vi "BuildExperiment.vi"(0 "object in":refnum<class "Experiment.lvclass">, 1 "List of Frequencies":dbl[](array[numeric]) min=0.001, 2 "List of Amplitudes":dbl[](array[numeric]) min=0.001, 3 "Number of Images":i32, 4 "wait time(s)":dbl, 5 "error in (no error)":errorcluster, 7 "Flow":dbl[](array[numeric])) -> (14 "object out":refnum<class "Experiment.lvclass">, 17 "# elements in queue":i32, 19 "error out":errorcluster)   [LabVIEW 2023, in "Experiment.lvclass"]
uses:
  Experiment.lvclass
  Experiment.lvclass/Experiment.ctl
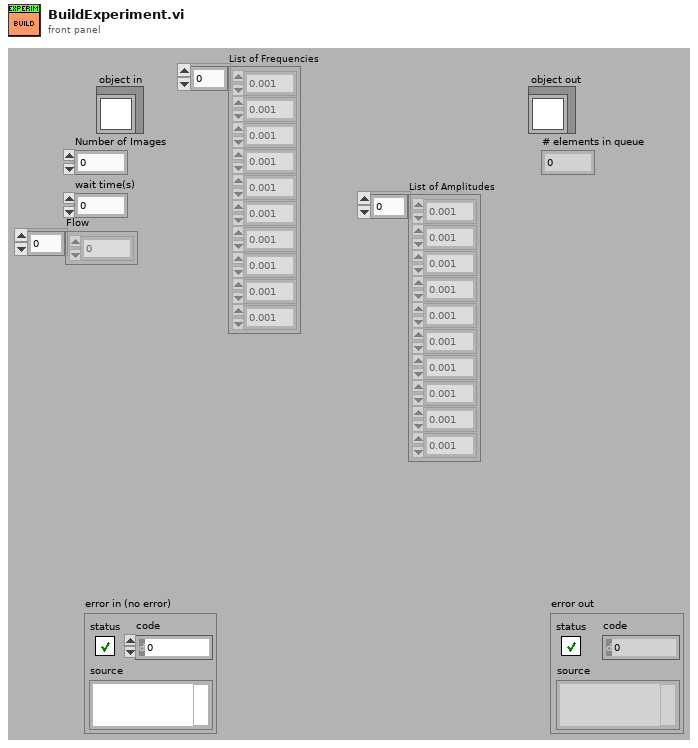
[diagram p1: front panel]
types:
  T1 = cluster{"index":i32, "Level(ml)":dbl, "Flow":dbl}
  T2 = cluster{"Enable Output WFG Ch1":bool, "Enable Output WFG Ch 2":bool}
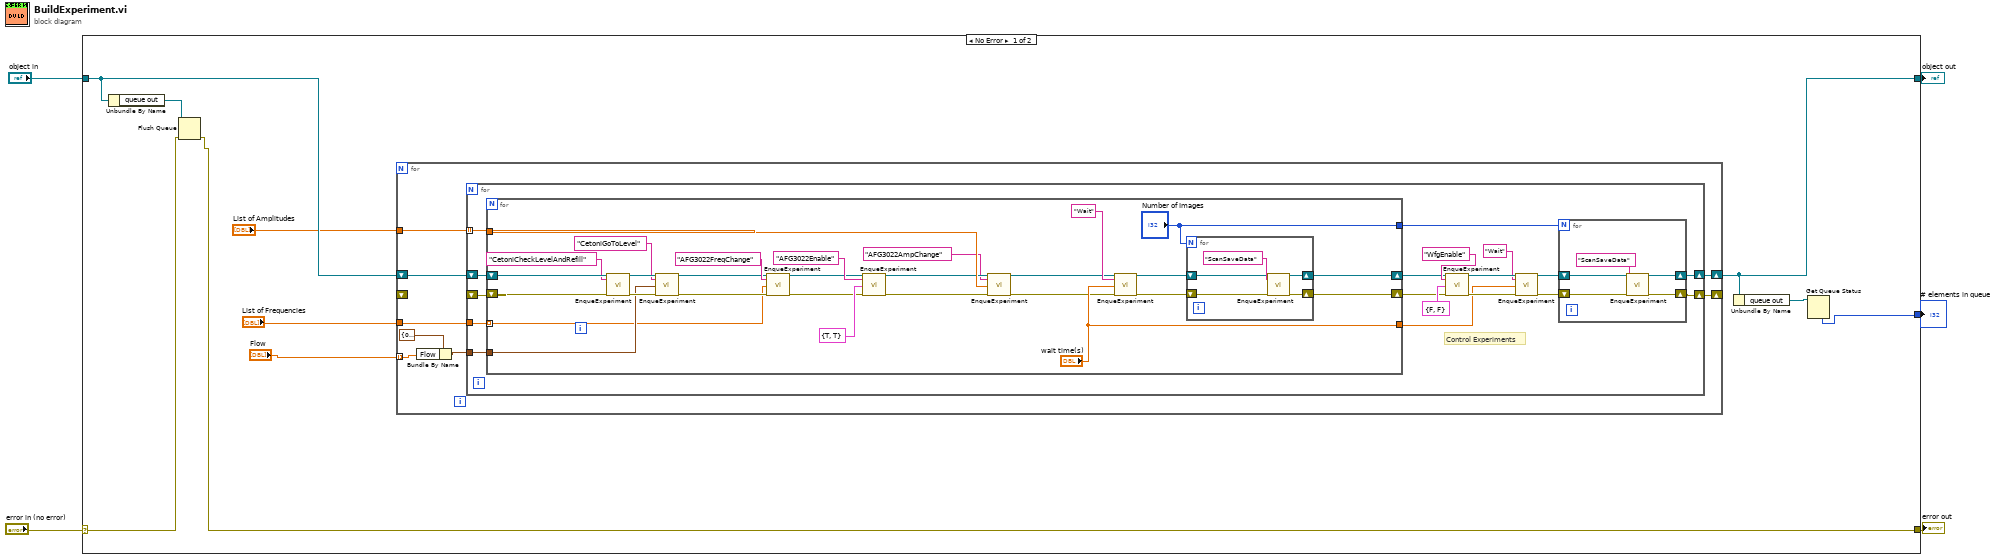
[diagram p0: block diagram]
diagram:
  n1 = case shown="No Error" "error in (no error)" {
    selector: "error in (no error)" -> [w12 w81]
    tunnel: [w11 w81] -> w4
    tunnel: [w10 w80] -> w2
    tunnel: "object in" -> [w14 w80]
    tunnel: [w8 _] -> w1
    frame No Error {
      n2 = Unbundle By Name(w14) -> ("queue out"=w13:refnum<queue>)
      n3 = Flush Queue(queue=w13, error in (no error)=w12) -> (error out=w11:errorcluster)  [unwired: 2 out]
      n4 = for {
        tunnel: "List of Frequencies" -> [w23]
        tunnel: "List of Amplitudes" -> [w20]
        shift-right: [w21] -> w10
        shift-left: w14 -> [w22]
        shift-right: [w19] -> _
        shift-left: _ -> [_]
        tunnel: "Flow" -> [w17] mode=indexing
        n5 = Bundle By Name(cluster=T1 {"index"=0, "Level(ml)"=0.0, "Flow"=0.0} ("GoToLevelSettings"), "Flow"=w17) -> (w16:T1)
        n6 = for {
          tunnel: w23 -> [w40]
          shift-right: [w31] -> w21
          shift-left: w22 -> [w39]
          tunnel: w20 -> [w41] mode=indexing
          tunnel: w16 -> [w25]
          shift-right: [w26] -> w19
          shift-left: _ -> [w24]
          # "Control Experiments"
          n7 = for {
            tunnel: w41 -> [w74]
            shift-right: [w65] -> w30
            shift-left: w39 -> [w63]
            tunnel: w40 -> [w50] mode=indexing
            tunnel: ["Number of Images"] -> w27
            shift-right: [w64] -> w28
            shift-left: w24 -> [w62]
            tunnel: ["wait time(s)"] -> w29
            tunnel: w25 -> [w56]
            n8 = call-dynamic "EnqueExperiment.vi"("object in"=w63, "Message"="CetoniCheckLevelAndRefill", "error in (no error)"=w62) -> ("object out"=w58:refnum<class "Experiment.lvclass">, "error out"=w60:errorcluster)  [unwired: 15 in]
            n9 = call-dynamic "EnqueExperiment.vi"("object in"=w58, "Message"="CetoniGoToLevel", "Message Data"=w56, "error in (no error)"=w60) -> ("object out"=w57:refnum<class "Experiment.lvclass">, "error out"=w59:errorcluster)  [unwired: 14 in]
            n10 = call-dynamic "EnqueExperiment.vi"("object in"=w57, "Message"="AFG3022FreqChange", "Message Data"=w50, "error in (no error)"=w59) -> ("object out"=w70:refnum<class "Experiment.lvclass">, "error out"=w68:errorcluster)  [unwired: 14 in]
            n11 = call-dynamic "EnqueExperiment.vi"("object in"=w70, "Message"="AFG3022Enable", "Message Data"=T2 {"Enable Output WFG Ch1"=TRUE, "Enable Output WFG Ch 2"=TRUE} ("OutputEnable 2"), "error in (no error)"=w68) -> ("object out"=w73:refnum<class "Experiment.lvclass">, "error out"=w67:errorcluster)  [unwired: 14 in]
            n12 = call-dynamic "EnqueExperiment.vi"("object in"=w73, "Message"="AFG3022AmpChange", "Message Data"=w74, "error in (no error)"=w67) -> ("object out"=w47:refnum<class "Experiment.lvclass">, "error out"=w48:errorcluster)  [unwired: 14 in]
            n13 = call-dynamic "EnqueExperiment.vi"("object in"=w47, "Message"="Wait", "Message Data"="wait time(s)", "error in (no error)"=w48) -> ("object out"=w54:refnum<class "Experiment.lvclass">, "error out"=w53:errorcluster)  [unwired: 14 in]
            n14 = for {
              N: "Number of Images" -> [_]
              shift-right: [w76] -> w65
              shift-left: w54 -> [w77]
              shift-right: [w75] -> w64
              shift-left: w53 -> [w78]
              n15 = call-dynamic "EnqueExperiment.vi"("object in"=w77, "Message"="ScanSaveData", "error in (no error)"=w78) -> ("object out"=w76:refnum<class "Experiment.lvclass">, "error out"=w75:errorcluster)  [unwired: 15 in]
            }
          }
          n16 = call-dynamic "EnqueExperiment.vi"("object in"=w30, "Message"="WfgEnable", "Message Data"=T2 {"Enable Output WFG Ch1"=FALSE, "Enable Output WFG Ch 2"=FALSE} ("OutputEnable 2"), "error in (no error)"=w28) -> ("object out"=w35:refnum<class "Experiment.lvclass">, "error out"=w37:errorcluster)  [unwired: 14 in]
          n17 = call-dynamic "EnqueExperiment.vi"("object in"=w35, "Message"="Wait", "Message Data"=w29, "error in (no error)"=w37) -> ("object out"=w36:refnum<class "Experiment.lvclass">, "error out"=w38:errorcluster)  [unwired: 14 in]
          n18 = for {
            N: w27 -> [_]
            shift-right: [w43] -> w26
            shift-left: w38 -> [w45]
            shift-right: [w42] -> w31
            shift-left: w36 -> [w44]
            n19 = call-dynamic "EnqueExperiment.vi"("object in"=w44, "Message"="ScanSaveData", "error in (no error)"=w45) -> ("object out"=w42:refnum<class "Experiment.lvclass">, "error out"=w43:errorcluster)  [unwired: 15 in]
          }
        }
      }
      n20 = Unbundle By Name(w10) -> ("queue out"=w9:refnum<queue>)
      n21 = Get Queue Status(queue=w9) -> (# elements in queue=w8:i32)  [unwired: 2 in, 7 out]
    }
    frame Error {
    }
  }
  "error out" <- w4
  "object out" <- w2
  "# elements in queue" <- w1
